vi "Read Part Fiducials.vi"(6 "Part Type":enum16{"HDI", "BBM", "HDI-on-BBM"}(ring), 7 "Dispose Images?":bool=TRUE, 8 "error in":errorcluster, 9 "Slot":i32, 10 "Chuck":i32, 11 "CameraTool in":refnum<class "CameraTool Class.lvclass">) -> (0 "error out":errorcluster, 2 "Fiducials":T3(array[cluster]), 3 "CameraTool out":refnum<class "CameraTool Class.lvclass">)   [LabVIEW 2011, in "CameraTool Class.lvclass"]
uses:
  CameraTool Class.lvclass
  Utils/Type Definitions/Physical Image.ctl
  Vec3d Class/Vec3d Class.lvclass
  <vilib>/vision/Image Controls.llb/IMAQ Image.ctl
  WorkTable Class/WorkTable Class.lvclass
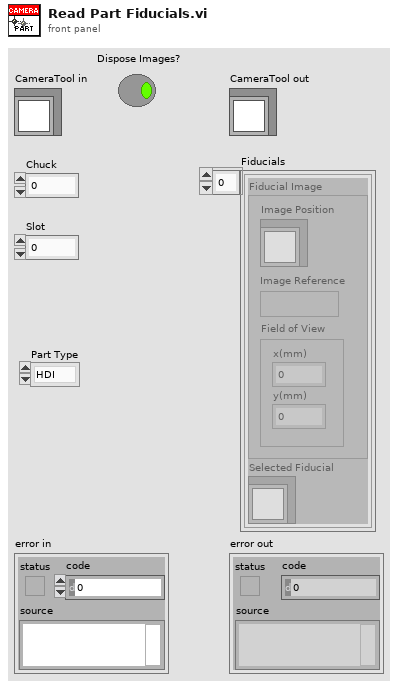
[diagram p1: front panel]
types:
  T1 = typedef "Physical Image.ctl" = cluster{"Image Position":refnum<class "Vec3d Class.lvclass">, "Image Reference":T2, "Field of View":cluster{"x(mm)":dbl, "y(mm)":dbl}}
  T2 = typedef "IMAQ Image.ctl" = refnum<image>
  T3 = cluster{"Fiducial Image":T1, "Selected Fiducial":refnum<class "Vec3d Class.lvclass">}[]
  T4 = cluster{"Fiducial Type":string, "Selection Criteria":enum16{"Single", "Top", "Bottom"}}
  T5 = typedef "Worktable_Module Slot.ctl" = cluster{"Slot State":enum16{"Empty", "Unglued", "Stamped", "PartOnTop", "Weighted", "Unpotted", "Potted"}, "BBM Type":enum16{"None", "BBM", "GlassSlide"}, "HDI Type":enum16{"None", "HDI", "Polyimide"}, "Vacuum Channel":u8, "Location/Orientation BBM":T6, "Location/Orientation HDI":T6, "S/N":string}
  T6 = typedef "Position_Orientation.ctl" = cluster{"Center":refnum<class "Vec3d Class.lvclass">, "Orientation":refnum<class "Orient3d Class.lvclass">}
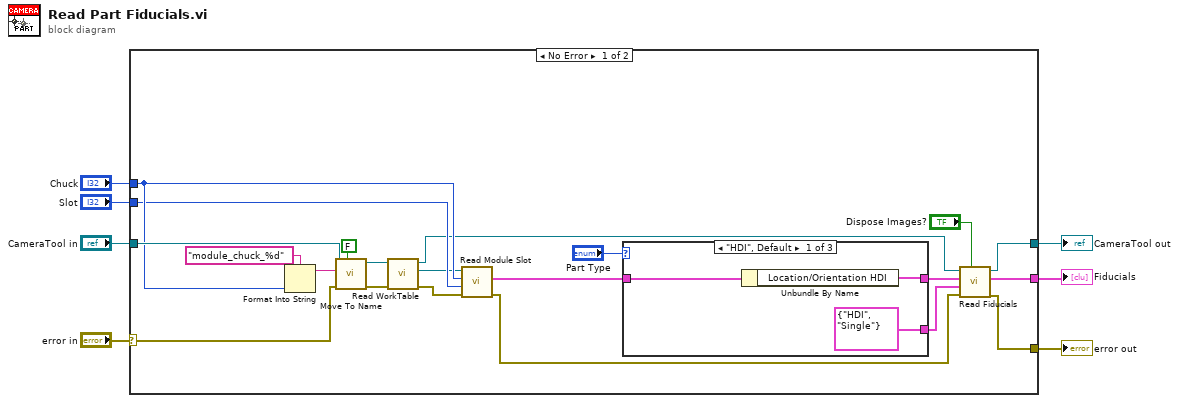
[diagram p0: block diagram]
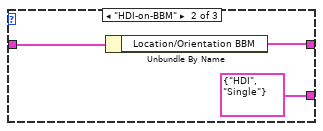
[diagram p2: hidden frame]
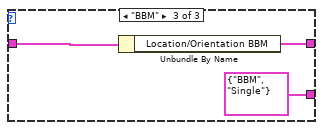
[diagram p3: hidden frame]
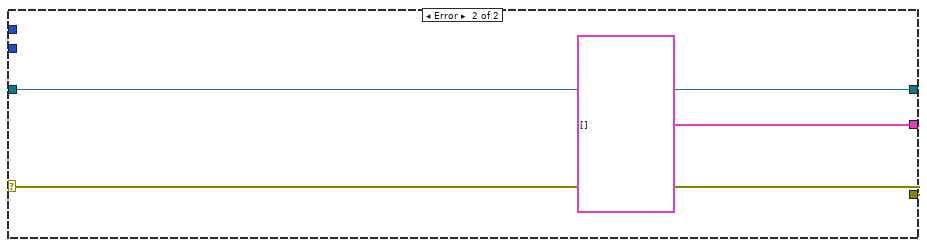
[diagram p4: hidden frame]
diagram:
  n1 = case shown="No Error" "error in" {
    selector: "error in" -> [w15 w40]
    tunnel: [w26 w40] -> w5
    tunnel: "CameraTool in" -> [w16 w39]
    tunnel: "Chuck" -> [w14 _]
    tunnel: "Slot" -> [w13 _]
    tunnel: [w28 w39] -> w2
    tunnel: [w25 T3 [] ("Fiducials")] -> w1
    frame No Error {
      n2 = Format Into String(format string="module_chuck_%d", w14) -> (resulting string=w18:string)  [unwired: 2 in, 1 out]
      n3 = call-dynamic "Move To Name.vi"("Move if Same"=FALSE, "error in"=w15, "Destination Name"=w18, "Gantry in"=w16) -> ("error out"=w22:errorcluster, "Gantry out"=w21:refnum<class "CameraTool Class.lvclass">)  [unwired: 6 in]
      n4 = call-dynamic "Read WorkTable.vi"("error in"=w22, "Gantry Class in"=w21) -> ("error out"=w20:errorcluster, "WorkTable Class.lvclass"=w11:refnum<class "WorkTable Class.lvclass">, "Gantry Class out"=w8:refnum<class "CameraTool Class.lvclass">)  [unwired: 7 in]
      n5 = call-dynamic "Read Module Slot.vi"("error in"=w20, "slot"=w13, "chuck"=w14, "WorkTable in"=w11) -> ("error out"=w9:errorcluster, "Module Slot"=w12:T5)  [unwired: 5 in, 1 out]
      n6 = case shown="\"HDI\", Default" "Part Type" {
        tunnel: [w29 w32 w37] -> w24
        tunnel: [T4 {"Fiducial Type"="HDI", "Selection Criteria"=enum."Single"} ("Fiducial Acquisition Parameters") T4 {"Fiducial Type"="HDI", "Selection Criteria"=enum."Single"} ("Fiducial Acquisition Parameters") T4 {"Fiducial Type"="BBM", "Selection Criteria"=enum."Single"} ("Fiducial Acquisition Parameters")] -> w23
        tunnel: w12 -> [w30 w33 w35]
        frame "HDI", Default {
          n7 = Unbundle By Name(w30) -> ("Location/Orientation HDI"=w29:T6)
        }
        frame "HDI-on-BBM" {
          n8 = Unbundle By Name(w33) -> ("Location/Orientation BBM"=w32:T6)
        }
        frame "BBM" {
          n9 = Unbundle By Name(w35) -> ("Location/Orientation BBM"=w37:T6)
        }
      }
      n10 = call-dynamic "Read Fiducials.vi"("Dispose Images?"="Dispose Images?", "error in"=w9, "Fiducial Acquisition Parameters"=w23, "Location/Orientation in"=w24, "CameraTool in"=w8) -> ("error out"=w26:errorcluster, "Fiducials"=w25:T3, "CameraTool out"=w28:refnum<class "CameraTool Class.lvclass">)  [unwired: 4 in]
    }
    frame Error {
    }
  }
  "CameraTool out" <- w2
  "error out" <- w5
  "Fiducials" <- w1
